vi "串口上位机.vi"() -> ()   [LabVIEW 2017]
uses:
  <vilib>/Instr/_visa.llb/VISA Configure Serial Port (Instr).vi
  <vilib>/Utility/file.llb/Read From Spreadsheet File (I64).vi
  <vilib>/Utility/file.llb/Write To Spreadsheet File (I64).vi
panel:
  out "元素":u8
  out "无符号字节数组":u8[](array[numeric])
  out "接收字节缓冲区":u8[](array[numeric])
  in  "选项卡控件":enum32{"帧采集", "采集信号", "信号回放"}(tab)
  out "?":bool
  in  "清空接收":bool
  in  "确定按钮":bool
  in  "?":bool
  out "时间：年月日-小时-分":string
  in  "保存数据格式":path=path "data.txt"
  in  "布尔 2":bool=TRUE
  in  "baud rate":u32=115200 caption="波特率"
  in  "VISA resource name":refnum<visa-resource-name>="COM1" caption="串口号"
  out "bytes read":u32=7 caption="读取的字节"
  in  "data bits":u16=8 caption="数据比特" min=5 max=8 step=1
  in  "parity":u16(ring) caption="奇偶" items=["无", "奇", "偶", "标记", "空格"]
  in  "stop bits":u16(ring)=10 caption="停止位" items=["1.0"=10, "1.5"=15, "2.0"=20]
  in  "flow control":u16(ring) caption="流程控制" items=["无"=0, "XON/XOFF"=1, "RTS/CTS"=2, "DTR/DSR"=4]
  in  "delay before read (ms)":u32=1 caption="读取前延时(ms)"
  out "波形显示":T1
  in  "布尔":bool
  in  "保存帧格式":path=path "frame.txt"
  in  "string to write 2":string="abcdefg\n" caption="写入字符串"
  out "还原后的数据":u32
  out "类型2":bool
  out "read string 2":string="*IDN?\n" caption="读取字符串"
  out "类型3":bool
  out "类型1":bool
  out "波形显示 2":u32[](graph) caption="波形显示"
  in  "数据位数":u16(ring)=8 items=["8"=8, "16"=16, "32"=32]
  in  "信号回放按键":bool
  out "波形显示 3":i64[][](graph) caption="波形显示"
  in  "数据格式文件":path=path "data.txt"
  # "1. 帧格式：\n    0xAA 类型 数据低字位 数据高字节 保留字节 保留字节 异或校验字节\n2. 类型： 0: nothing 1: 声方向 2: 目标类型 3: 过零率\n3. 此处无浏览按钮的路径都使用当前VI的相对路径"
  # "注：数据先低字节后高字节"
  # "1. 回放的信号文件必须是数据格式存储的文件\n2. 此处使用绝对路径"
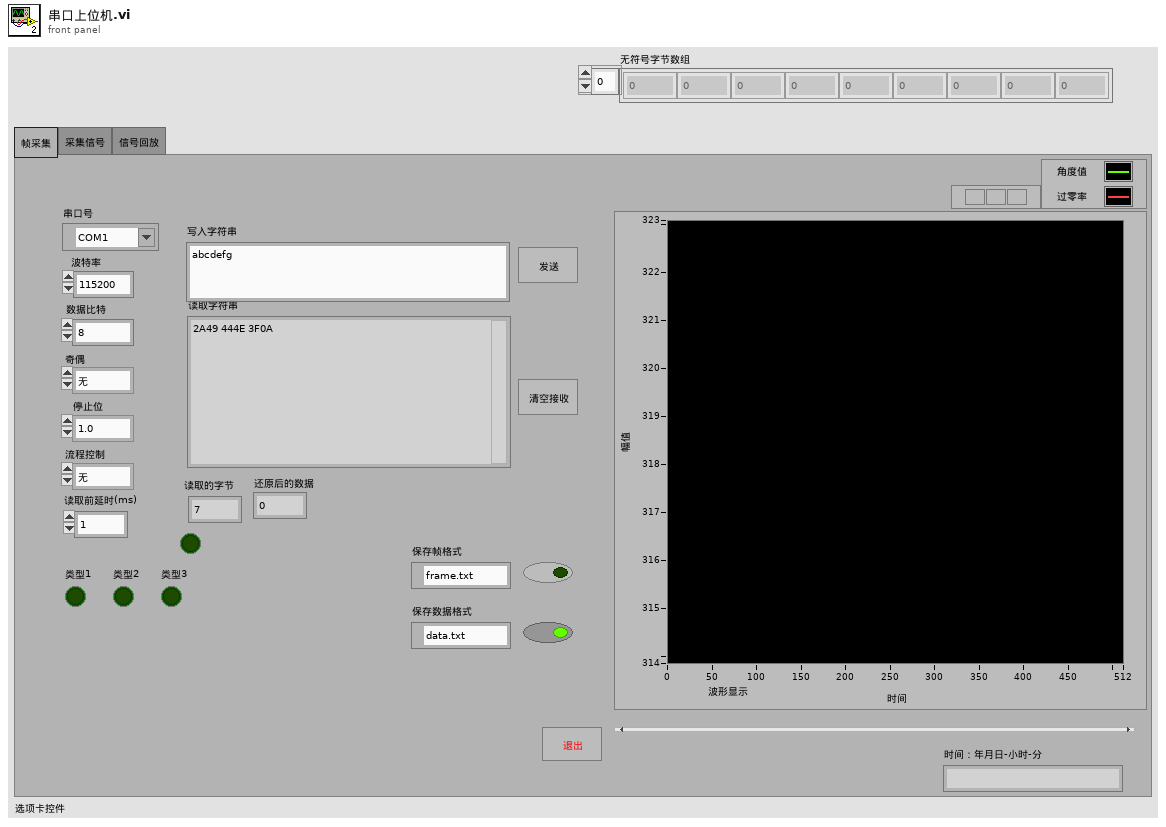
[diagram p1: front panel]
types:
  T1 = typedef "控件 1.ctl" = cluster{u32, u32}
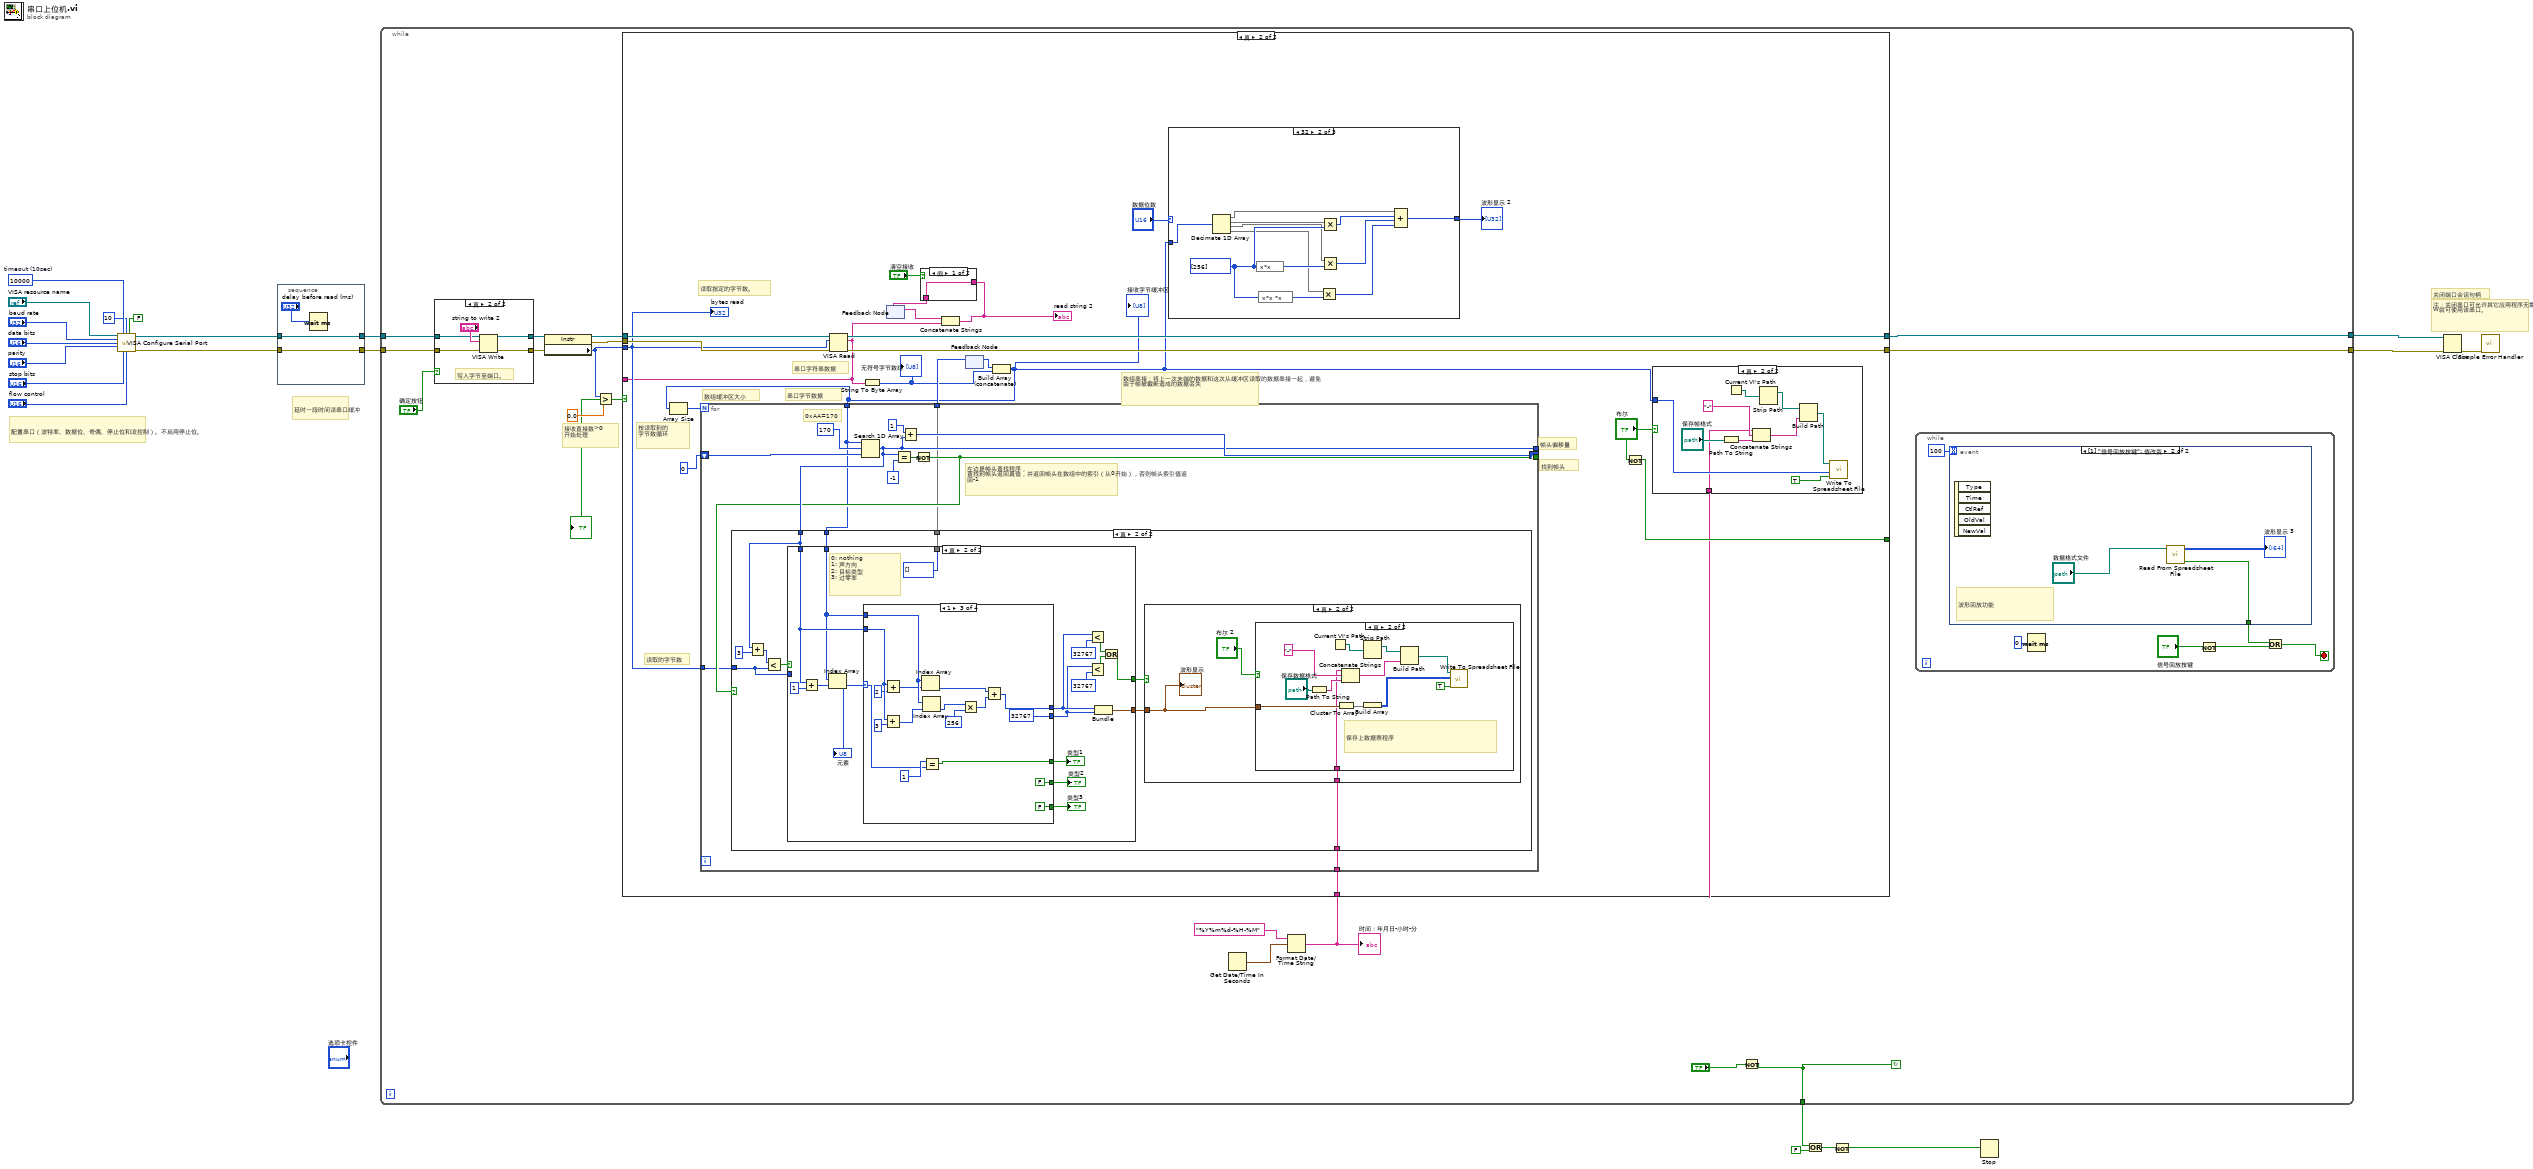
[diagram p0: block diagram]
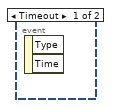
[diagram p3: hidden frame]
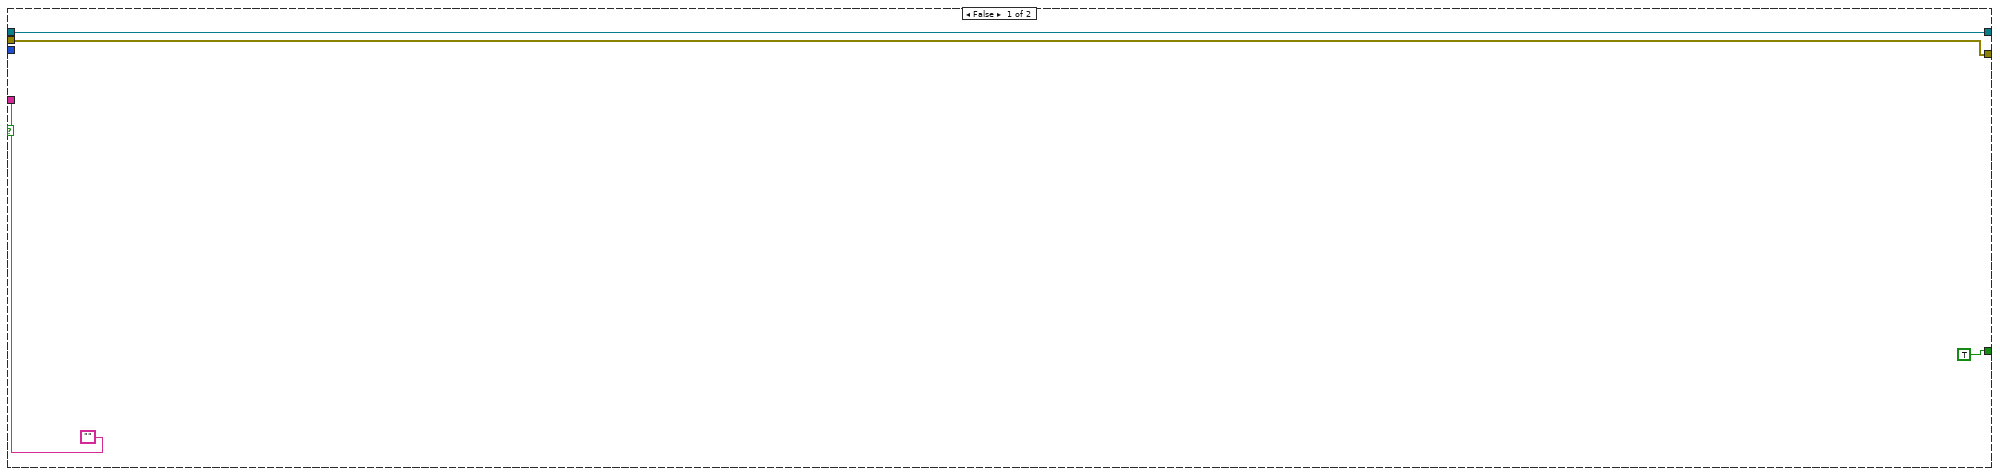
[diagram p4: hidden frame]
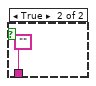
[diagram p5: hidden frame]
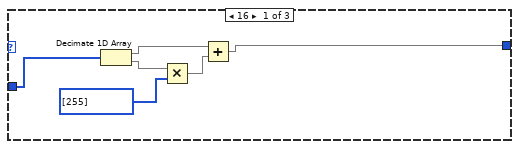
[diagram p6: hidden frame]
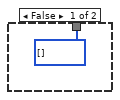
[diagram p9: hidden frame]
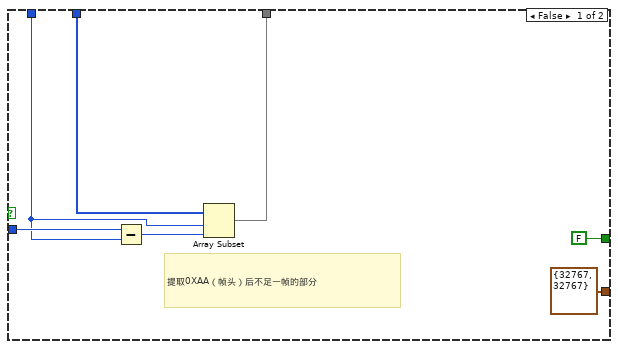
[diagram p10: hidden frame]
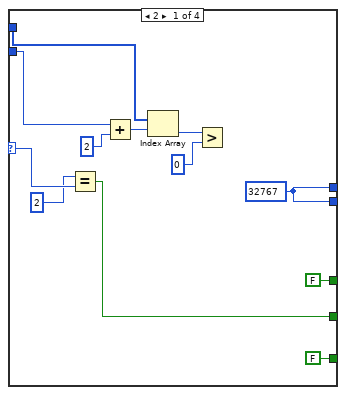
[diagram p11: hidden frame]
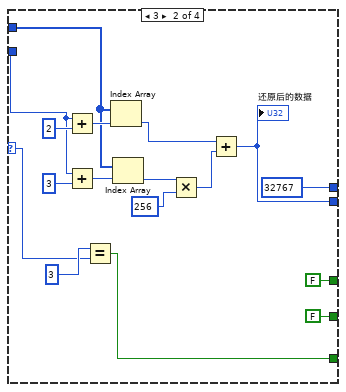
[diagram p12: hidden frame]
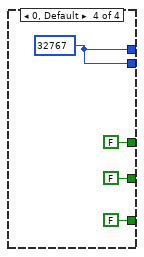
[diagram p13: hidden frame]
diagram:
  w8 = u32 10000  # timeout (10sec)
  # "延时一段时间读串口缓冲"
  # "配置串口（波特率、数据位、奇偶、停止位和流控制）。不启用停止位。"
  # "注：关闭串口可允许其它应用程序无需退出LabVIEW就可使用该串口。"
  # "关闭端口会话句柄"
  n1 = call-poly "VISA Configure Serial Port"("VISA resource name"="VISA resource name", "timeout (10sec)"=w8, "termination char\n(0xA = '\\n' = LF)"=u8 10 ("termination char\n(0xA = '\\n' = LF)"), "Enable Termination\nChar (T)"=FALSE ("Enable Termination\nChar (T)"), "baud rate (9600)"="baud rate", "data bits (8)"="data bits", "parity (0:none)"="parity", "stop bits (10: 1 bit)"="stop bits", "flow control (0:none)"="flow control") -> ("VISA resource name out"=w2:refnum<visa-resource-name>, "error out"=w1:errorcluster)  [unwired: 1 in, 4 out]
  n2 = stacked-sequence {
    tunnel: w1 -> [w23]
    tunnel: [w23] -> w17
    tunnel: w2 -> [w22]
    tunnel: [w22] -> w16
    frame #0 {
      n3 = Wait (ms)(milliseconds to wait="delay before read (ms)") -> ()  [unwired: 1 out]
    }
  }
  n4 = while {
    tunnel: [w40] -> w20
    tunnel: [w39] -> w19
    tunnel: w17 -> [w28]
    tunnel: w16 -> [w30]
    tunnel: [w25] -> w14
    stop <- w25 continue-if-true
    # "接收直接数>0\n开始处理"
    n5 = case shown="真" "确定按钮" {
      tunnel: [w42 w47] -> w27
      tunnel: w30 -> [w41 w45]
      tunnel: w28 -> [w42 w44]
      tunnel: [w41 w43] -> w29
      frame False {
      }
      frame True {
        # "写入字节至端口。"
        n6 = VISA Write(VISA resource name=w45, write buffer="string to write 2", error in (no error)=w44) -> (VISA resource name out=w43:refnum<visa-resource-name>, error out=w47:errorcluster)  [unwired: 1 out]
      }
    }
    n7 = property class="Instr"(reference=w29, error in=w27) -> (reference out=w38:refnum<visa-resource-name>, error out=w37:errorcluster, "Serial Settings:Number of Bytes at Serial Port"=w35:u32)
    n8 = Greater?(x=w35, y=0.0) -> (0:w34:bool)
    "?" <- w34
    n9 = Get Date/Time In Seconds() -> (seconds since 1Jan1904=w33:timestamp)
    n10 = Format Date/Time String(time format string (%c)="%Y%m%d-%H-%M" ("时间格式字符串(%c)"), seconds (now)=w33) -> (date/time string=w31:string)  [unwired: 1 in]
    "时间：年月日-小时-分" <- w31
    n11 = case shown="真" w34 {
      tunnel: [w58 w81] -> w40
      tunnel: [w59 w78] -> w39
      tunnel: w38 -> [w59 w80]
      tunnel: w37 -> [w58 w79]
      tunnel: w35 -> [_ w73]
      tunnel: ["" w64] -> _
      tunnel: [TRUE w75] -> _
      tunnel: w31 -> [_ w74]
      frame False {
      }
      frame True {
        # "串口字符串数据"
        # "串口字节数据"
        # "按读取到的\n字节数循环"
        # "数组串接：将上一次末端的数据和这次从缓冲区读取的数据串接一起，避免由于帧被截断造成的数据丢失"
        # "读取的字节数"
        # "数组缓冲区大小"
        # "找到帧头"
        # "帧头偏移量"
        # "读取指定的字节数。"
        n12 = VISA Read(VISA resource name=w80, byte count=w73, error in (no error)=w79) -> (VISA resource name out=w78:refnum<visa-resource-name>, read buffer=w64:string, error out=w81:errorcluster)  [unwired: 1 out]
        n13 = String To Byte Array ("字符串转字节函数")(string=w64) -> (unsigned byte array=w71:u8[])
        "无符号字节数组" <- w71
        n14 = feedback #1() -> (w65:string)  [unwired: 1 in]
        n15 = Concatenate Strings(w65, w64) -> (w62:string)
        "read string 2" <- w62
        n16 = case shown="假" "清空接收" {
          tunnel: w62 -> [w82 _]
          tunnel: [w82 ""] -> w61
          frame False {
          }
          frame True {
          }
        }
        n17 = feedback-in #1(w61) -> ()
        n18 = feedback #2() -> (w70:u8[])  [unwired: 1 in]
        n19 = Build Array (concatenate)(w70, w71) -> (w66:u8[])
        "接收字节缓冲区" <- w66
        n20 = Array Size(array=w66) -> (size(s)=w69:i32)
        n21 = for {
          N: w69 -> [_]
          shift-right: [w121] -> _
          shift-left: 0 -> [w123]
          tunnel: [w118] -> _
          tunnel: [w117] -> _
          tunnel: w66 -> [w116]
          tunnel: w74 -> [w115]
          tunnel: w73 -> [w114]
          tunnel: [w113] -> w72
          # "左边是帧头查找程序，\n查找到帧头返回真值，并返回帧头在数组中的索引（从0开始），否则帧头索引值返回-1"
          # "0xAA=170"
          n22 = Search 1D Array(1D array=w116, element=u8 170 ("元素"), start index (0)=w123) -> (index of element=w118:i32)
          n23 = Equal?(x=w118, y=-1) -> (x = y?=w119:bool)
          n24 = Add(x=1, y=w118) -> (x+y=w121:i32)
          n25 = Not(x=w119) -> (.not. x?=w117:bool)
          n26 = case shown="真" w117 {
            tunnel: w118 -> [_ w127]
            tunnel: w116 -> [_ w135]
            tunnel: w115 -> [_ w132]
            tunnel: w114 -> [_ w128]
            tunnel: [u8[] [] w126] -> w113
            frame False {
            }
            frame True {
              n27 = Add(x=w127, y=u32 3) -> (x+y=w129:u32)
              n28 = Less?(x=w129, y=w128) -> (x < y?=w130:bool)
              n29 = case shown="真" w130 {
                tunnel: w127 -> [w138 w157]
                tunnel: w135 -> [w137 w156]
                tunnel: [cluster{u32, u32} {32767, 32767} w153] -> w134
                tunnel: [FALSE w147] -> w133
                tunnel: w128 -> [w140 _]
                tunnel: [w136 u8[] []] -> w126
                frame False {
                  # "提取0XAA（帧头）后不足一帧的部分"
                  n30 = Subtract(x=w140, y=w138) -> (x-y=w139:u32)
                  n31 = Array Subset(array=w137, index=w138, length=w139) -> (w136:u8[])
                }
                frame True {
                  # "0: nothing\n1: 声方向\n2: 目标类型\n3: 过零率"
                  n32 = Add(x=w157, y=u8 1) -> (x+y=w158:i32)
                  n33 = Index Array(array=w156, index=w158) -> (element=w155:u8)
                  "元素" <- w155
                  n34 = case shown="1" w155 {
                    selector: w155 -> [w164 w175 w192 _]
                    tunnel: w157 -> [w171 w186 w205 _]
                    tunnel: w156 -> [w168 w183 w204 _]
                    tunnel: [w165 u32 32767 w195 w209] -> w151
                    tunnel: [w165 w178 u32 32767 w209] -> w150
                    tunnel: [FALSE FALSE w191 FALSE] -> w145
                    tunnel: [w161 FALSE FALSE FALSE] -> w144
                    tunnel: [FALSE w172 FALSE FALSE] -> w143
                    frame 2 {
                      w165 = u32 32767
                      n35 = Equal?(x=2 ("y"), y=w164) -> (x = y?=w161:bool)
                      n36 = Add(x=w171, y=2) -> (x+y=w169:i32)
                      n37 = Index Array(array=w168, index=w169) -> (element=w167:u8)
                      n38 = Greater?(x=w167, y=u8 0) -> ()  [unwired: 1 out]
                    }
                    frame 3 {
                      n39 = Add(x=w186, y=2) -> (x+y=w187:i32)
                      n40 = Add(x=w186, y=3) -> (x+y=w184:i32)
                      n41 = Equal?(x=3 ("y"), y=w175) -> (x = y?=w172:bool)
                      n42 = Index Array(array=w183, index=w187) -> (element=w179:u8)
                      n43 = Index Array(array=w183, index=w184) -> (element=w182:u8)
                      n44 = Multiply(x=w182, y=u32 256) -> (x*y=w180:u32)
                      n45 = Add(x=w179, y=w180) -> (x+y=w178:u32)
                      "还原后的数据" <- w178
                    }
                    frame 1 {
                      n46 = Add(x=w205, y=3 ("索引")) -> (x+y=w198:i32)
                      n47 = Add(x=w205, y=2 ("索引")) -> (x+y=w201:i32)
                      n48 = Index Array(array=w204, index=w201) -> (element=w203:u8)
                      n49 = Index Array(array=w204, index=w198) -> (element=w197:u8)
                      n50 = Equal?(x=1 ("y"), y=w192) -> (x = y?=w191:bool)
                      n51 = Multiply(x=w197, y=u32 256 ("x")) -> (x*y=w202:u32)
                      n52 = Add(x=w203, y=w202) -> (x+y=w195:u32)
                    }
                    frame 0, Default {
                      w209 = u32 32767
                    }
                  }
                  "类型1" <- w145
                  "类型2" <- w144
                  "类型3" <- w143
                  n53 = Less?(x=w151, y=u32 32767) -> (x < y?=w148:bool)
                  n54 = Less?(x=w150, y=u32 32767) -> (x < y?=w149:bool)
                  n55 = Bundle(w151, w150) -> (w153:cluster{u32, u32})  [unwired: 1 in]
                  n56 = Or(x=w148, y=w149) -> (x .or. y?=w147:bool)
                }
              }
              n57 = case shown="真" w133 {
                tunnel: w134 -> [_ w210]
                tunnel: w132 -> [_ w211]
                frame False {
                }
                frame True {
                  n58 = case shown="真" "布尔 2" {
                    tunnel: w210 -> [_ w223]
                    tunnel: w211 -> [_ w214]
                    frame False {
                    }
                    frame True {
                      # "保存上数据表程序"
                      n59 = Path To String(path="保存数据格式") -> (string=w216:string)
                      n60 = Current VI's Path() -> (path=w220:path)
                      n61 = Cluster To Array(cluster=w223) -> (array=w222:u32[])
                      n62 = Concatenate Strings(w214, "-" ("字符串"), w216) -> (w213:string)
                      n63 = Strip Path(path=w220) -> (stripped path=w219:path)  [unwired: 1 out]
                      n64 = Build Array(w222) -> (w221:u32[][])
                      n65 = Build Path(base path=w219, name or relative path=w213) -> (appended path=w218:path)
                      n66 = call-poly <vilib>:"Write To Spreadsheet File.vi"("append to file? (new file:F)"=TRUE, "2D data"=w221, "file path (dialog if empty)"=w218) -> ()  [unwired: 5 in, 1 out]
                    }
                  }
                  "波形显示" <- w210
                }
              }
            }
          }
        }
        n67 = feedback-in #2(w72) -> ()
        n68 = case shown="32" "数据位数" {
          tunnel: [w84 w90 w102] -> w67
          tunnel: w66 -> [w89 w101 w102]
          frame 16 {
            n69 = Decimate 1D Array(w89) -> (w85:u8[], w88:u8[])
            n70 = Multiply(x=w88, y=u8[] [255]) -> (x*y=w86:u8[])
            n71 = Add(x=w85, y=w86) -> (x+y=w84:u8[])
          }
          frame 32 {
            w97 = u32[] [256] ("y")
            n72 = Decimate 1D Array(w101) -> (w94:u8[], w100:u8[], w96:u8[], w95:u8[])
            n73 = expression code="x*x"(w97) -> (w99:u32[])
            n74 = expression code="x*x *x"(w97) -> (w98:u32[])
            n75 = Multiply(x=w95, y=w98) -> (x*y=w91:u32[])
            n76 = Multiply(x=w100, y=w97) -> (x*y=w93:u32[])
            n77 = Multiply(x=w96, y=w99) -> (x*y=w92:u32[])
            n78 = Compound Arithmetic op=ADD(w94, w93, w92, w91) -> (w90:u32[])
          }
          frame 8, Default {
          }
        }
        "波形显示 2" <- w67
        n79 = Not(x="布尔") -> (.not. x?=w75:bool)
        n80 = case shown="真" "布尔" {
          tunnel: w66 -> [_ w112]
          tunnel: w74 -> [_ w104]
          frame False {
          }
          frame True {
            n81 = Path To String(path="保存帧格式") -> (string=w106:string)
            n82 = Current VI's Path() -> (path=w110:path)
            n83 = Concatenate Strings(w104, "-" ("字符串"), w106) -> (w103:string)
            n84 = Strip Path(path=w110) -> (stripped path=w109:path)  [unwired: 1 out]
            n85 = Build Path(base path=w109, name or relative path=w103) -> (appended path=w108:path)
            n86 = call-poly <vilib>:"Write To Spreadsheet File.vi"("append to file? (new file:F)"=TRUE, "1D data"=w112, "file path (dialog if empty)"=w108) -> ()  [unwired: 5 in, 1 out]
          }
        }
        "bytes read" <- w73
      }
    }
    n87 = Not(x="?") -> (.not. x?=w25:bool)
    n88 = while {
      stop <- w48 stop-if-true
      n89 = event shown="[1] \"信号回放按键\": 值改变" {
        selector: _ -> [_ _]
        dyn-events: _ -> [_ _]
        timeout: 100 -> [_ _]
        tunnel: [_ w55] -> w50
        event Timeout {
          n90 = event-data() -> ()  [unwired: 1 in, 2 out]
        }
        event "信号回放按键": Value Change {
          # "波形回放功能"
          n91 = event-data() -> ()  [unwired: 1 in, 5 out]
          n92 = call-poly <vilib>:"Read From Spreadsheet File.vi"("file path (dialog if empty)"="数据格式文件") -> ("EOF?"=w55:bool, "all rows"=→"波形显示 3":i64[][])  [unwired: 6 in, 3 out]
        }
      }
      n93 = Wait (ms)(milliseconds to wait=u32 0 ("等待时间（毫秒）")) -> ()  [unwired: 1 out]
      n94 = Not(x="信号回放按键") -> (.not. x?=w49:bool)
      n95 = Or(x=w50, y=w49) -> (x .or. y?=w48:bool)
    }
  }
  n96 = Or(x=w14, y=FALSE) -> (x .or. y?=w15:bool)
  n97 = Not(x=w15) -> (.not. x?=w12:bool)
  n98 = Stop(stop? (T)=w12) -> ()
  n99 = VISA Close(VISA resource name=w19, error in (no error)=w20) -> (error out=w18:errorcluster)
  n100 = call <vilib>:"Simple Error Handler.vi"("error in (no error)"=w18) -> ()  [unwired: 1 in, 8 out]
